vi "Execute.vi"(8 "Error Input":errorcluster, 9 "FunctionCall":T1, 10 "SessionId":string, 11 "LiteAgent In":T2) -> (0 "Error Output":errorcluster, 2 "ToolReturn":cluster{"id":string, "result":variant}, 3 "LiteAgent Out":T2)   [LabVIEW 2017]
uses:
  C:/Users/Jan/Projects/LiteAgentSDK-LabVIEW/Source/Bin/LiteAgentSDK.LabVIEW.dll
  Source/Bin/LiteAgentSDK.LabVIEW.dll
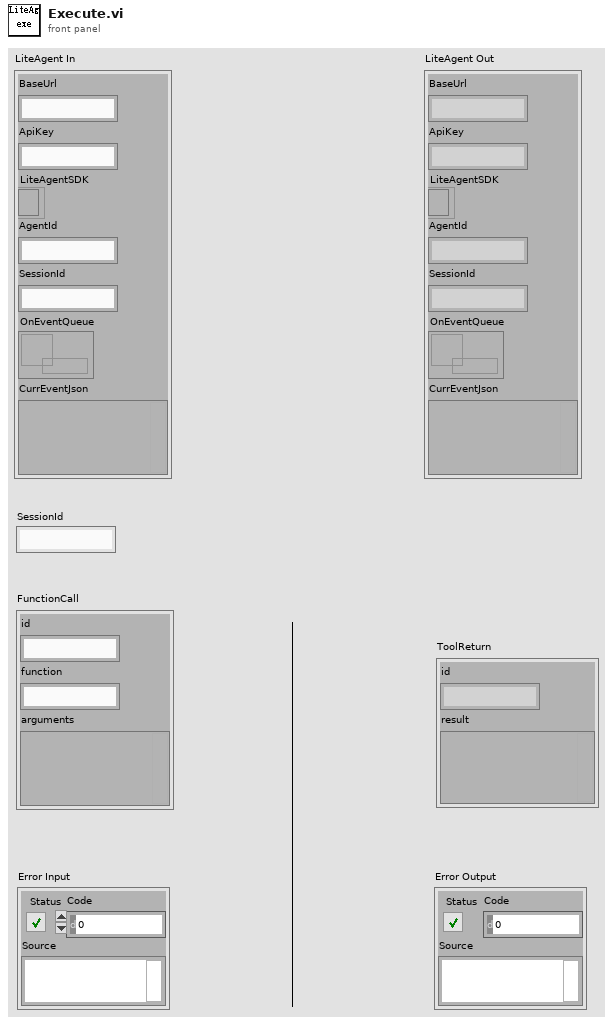
[diagram p1: front panel]
types:
  T1 = cluster{"id":string, "function":string, "arguments":variant}
  T2 = cluster{"BaseUrl":string, "ApiKey":string, "LiteAgentSDK":refnum<k24>, "AgentId":string, "SessionId":string, "OnEventQueue":refnum<queue>, "CurrEventJson":variant}
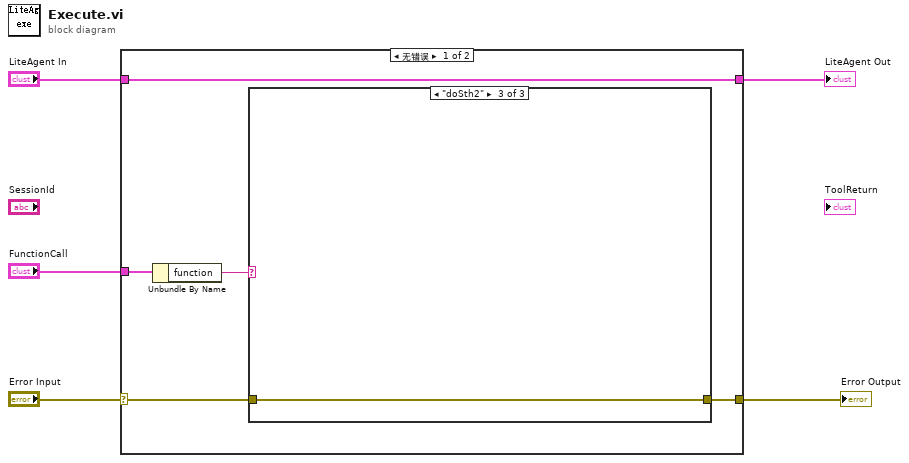
[diagram p0: block diagram]
diagram:
  n1 = case shown="无错误" "Error Input" {
    selector: "Error Input" -> [w9 w15]
    tunnel: [w6 w15] -> w4
    tunnel: "LiteAgent In" -> [w10 w14]
    tunnel: [w10 w14] -> w2
    tunnel: "FunctionCall" -> [w8 _]
    frame No Error {
      n2 = Unbundle By Name(w8) -> ("function"=w7:string)
      n3 = case shown="\"doSth2\"" w7 {
        tunnel: w9 -> [w11 w12 w13]
        tunnel: [w11 w12 w13] -> w6
        frame "\u0000", Default {
        }
        frame "doSth1" {
        }
        frame "doSth2" {
        }
      }
    }
    frame Error {
    }
  }
  "Error Output" <- w4
  "LiteAgent Out" <- w2
